vi "GPS .vi"(8 "滑动杆":i16(slide)=12 scale=0.0..18.0, 10 "纬度":string, 11 "经度":string) -> (2 "url":string)   [LabVIEW 2018]
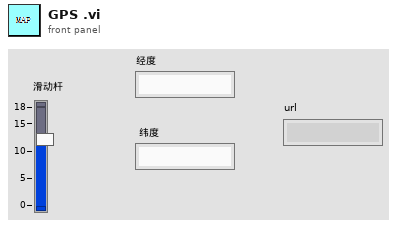
[diagram p1: front panel]
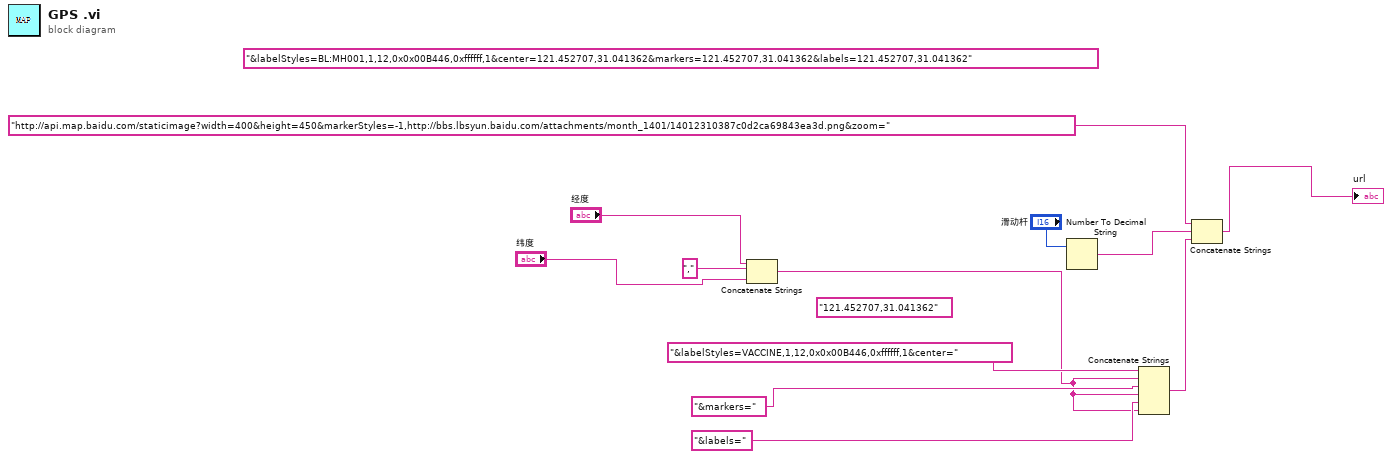
[diagram p0: block diagram]
diagram:
  (unwired) "121.452707,31.041362"
  (unwired) "&labelStyles=BL:MH001,1,12,0x0x00B446,0xffffff,1&center=121.452707,31.041362&markers=121.452707,31.041362&labels=121.452707,31.041362" ("连接的字符串")
  n1 = Concatenate Strings("经度", ",", "纬度") -> (w4:string)
  n2 = Number To Decimal String(number="滑动杆") -> (decimal integer string=w10:string)  [unwired: 1 in]
  n3 = Concatenate Strings("&labelStyles=VACCINE,1,12,0x0x00B446,0xffffff,1&center=", w4, "&markers=", w4, "&labels=", w4) -> (w5:string)
  n4 = Concatenate Strings("http://api.map.baidu.com/staticimage?width=400&height=450&markerStyles=-1,http://bbs.lbsyun.baidu.com/attachments/month_1401/14012310387c0d2ca69843ea3d.png&zoom=", w10, w5) -> (→"url":string)
